vi "Check If Pixels Belong In Sector.vi"() -> (3 "FIFO Timeout?":bool)   [LabVIEW 2013]
uses:
  Single Sector Pixel Cluster.ctl
  Globals/Sector Parameter Global.vi
  Globals/Pixel Location Global.vi
  <vilib>/rvi/FIFO/Fifo_Resource/nirvififoEmulationReadFpgaImpl.vi
  <vilib>/rvi/DataTransferAndStorage/Container/Common/niFpgaContainerGetUniqueNameForEmu.vi
  <vilib>/rvi/FIFO/Fifo_Resource/nirvififoEmulationWriteFpgaImpl.vi
  <vilib>/rvi/DataTransferAndStorage/Container/XNode/niFpgaContainer.xnode
  <vilib>/rvi/FIFO/Fifo_Resource/nirvififoEmulationRead.vi
  <vilib>/rvi/FIFO/Fifo_Resource/nirvififoEmulationWrite.vi
panel:
  out "End of  Data?":bool
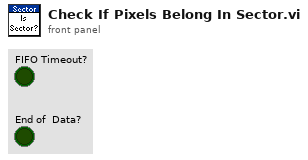
[diagram p1: front panel]
types:
  T1 = typedef "Single Sector Pixel Cluster.ctl" = cluster{"Sector #":u8, "Pixel Value":u8}
  T2 = typedef "Sector Parameter Cluster.ctl" = cluster{"Start Angle":fxp<+/-,17,2>, "End Angle":fxp<+/-,17,2>, "Inner Radius":u16, "Outter Radius":u16, "Hinge X":u16, "Hinge Y":u16, "NumWingSectors":u8}
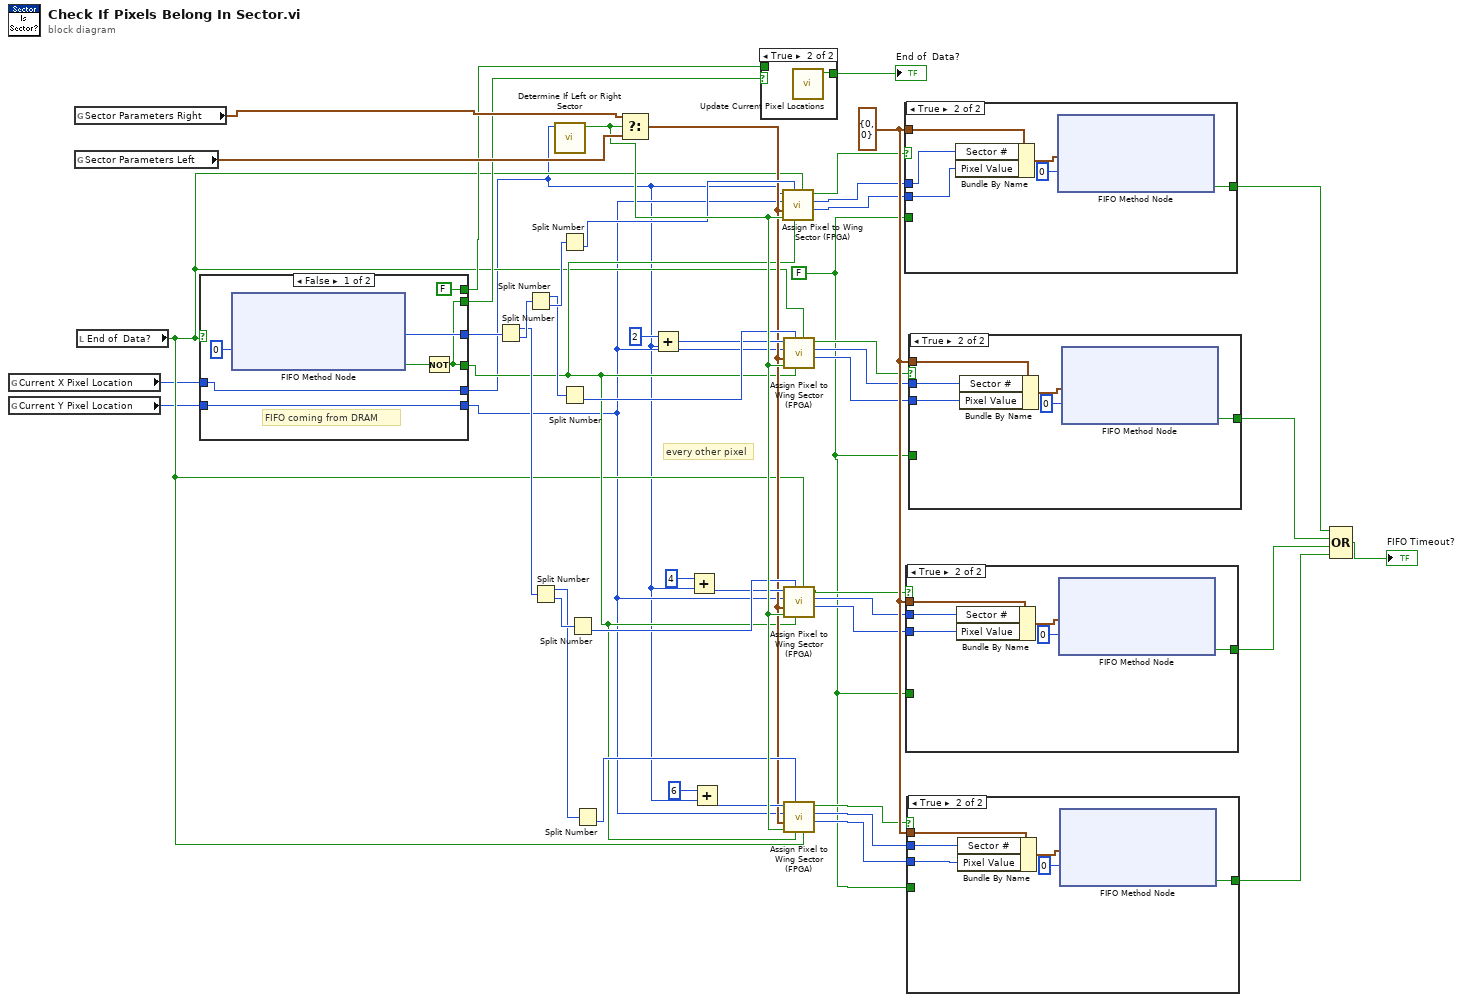
[diagram p0: block diagram]
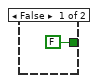
[diagram p3: hidden frame]
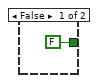
[diagram p4: hidden frame]
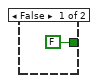
[diagram p5: hidden frame]
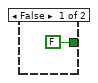
[diagram p6: hidden frame]
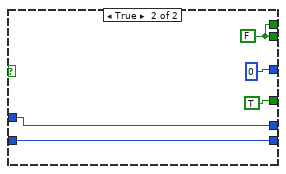
[diagram p7: hidden frame]
diagram:
  w27 = FALSE
  w40 = T1 {"Sector #"=0, "Pixel Value"=0} ("Single Sector Pixel")
  # "every other pixel"
  n1 = global read "Pixel Location Global.vi" "Current X Pixel Location"() -> (w1:u16)
  n2 = global read "Pixel Location Global.vi" "Current Y Pixel Location"() -> (w3:u16)
  n3 = global read "Sector Parameter Global.vi" "Sector Parameters Right"() -> (w47:T2)
  n4 = global read "Sector Parameter Global.vi" "Sector Parameters Left"() -> (w46:T2)
  n5 = local read "End of  Data?"() -> (w5:bool)
  n6 = case shown="False" w5 {
    tunnel: [w53 TRUE ("Timed Out?")] -> w8
    tunnel: [w55 u64 0 ("Element")] -> w45
    tunnel: [w53 w59] -> w7
    tunnel: [FALSE ("Timed Out?") w59] -> w6
    tunnel: [w51 w57] -> w4
    tunnel: w3 -> [w51 w57]
    tunnel: [w50 w58] -> w2
    tunnel: w1 -> [w50 w58]
    frame False {
      # "FIFO coming from DRAM"
      n7 = xnode ("FIFO Method Node")("Timeout"=0) -> ("Element"=w55:u64, "Timed Out?"=w54:bool)  [unwired: 1 in, 1 out]
      n8 = Not(x=w54) -> (.not. x?=w53:bool)
    }
    frame True {
      w59 = FALSE ("Timed Out?")
    }
  }
  n9 = Split Number(x=w45) -> (hi(x)=w25:u32, lo(x)=w26:u32)
  n10 = Split Number(x=w26) -> (hi(x)=w23:u16, lo(x)=w24:u16)
  n11 = Split Number(x=w25) -> (hi(x)=w21:u16, lo(x)=w22:u16)
  n12 = call "Determine If Left or Right Sector.vi"("X Pixel Location"=w2) -> ("Right Sector?"=w20:bool)  [unwired: 10 in]
  n13 = Split Number(x=w24) -> (lo(x)=w19:u8)  [unwired: 1 out]
  n14 = Split Number(x=w23) -> (lo(x)=w18:u8)  [unwired: 1 out]
  n15 = Split Number(x=w22) -> (lo(x)=w17:u8)  [unwired: 1 out]
  n16 = Split Number(x=w21) -> (lo(x)=w16:u8)  [unwired: 1 out]
  n17 = Select(t=w47, s=w20, f=w46) -> (s? t:f=w9:T2)
  n18 = Add(x=u16 2, y=w2) -> (x+y=w12:u16)
  n19 = Add(x=u16 4, y=w2) -> (x+y=w11:u16)
  n20 = Add(x=u16 6, y=w2) -> (x+y=w10:u16)
  n21 = case shown="True" w7 {
    tunnel: [w62 w63] -> w49
    tunnel: w6 -> [w62 _]
    frame False {
    }
    frame True {
      n22 = call "Update Current Pixel Locations.vi"() -> ("End of data?"=w63:bool)  [unwired: 11 in]
    }
  }
  "End of  Data?" <- w49
  n23 = call "Assign Pixel to Wing Sector (FPGA).vi"("End of Data?"=w5, "Valid Data?"=w8, "Pixel Intensity In"=w19, "Right Wing?"=w20, "Sector Parameters"=w9, "Pixel Y"=w4, "Pixel X"=w2) -> ("Pixel Intensity Out"=w37:u8, "sector #"=w38:u8, "output valid"=w39:bool)  [unwired: 2 out]
  n24 = call "Assign Pixel to Wing Sector (FPGA).vi"("End of Data?"=w5, "Valid Data?"=w8, "Pixel Intensity In"=w18, "Right Wing?"=w20, "Sector Parameters"=w9, "Pixel Y"=w4, "Pixel X"=w12) -> ("Pixel Intensity Out"=w34:u8, "sector #"=w35:u8, "output valid"=w36:bool)  [unwired: 2 out]
  n25 = call "Assign Pixel to Wing Sector (FPGA).vi"("End of Data?"=w5, "Valid Data?"=w8, "Pixel Intensity In"=w17, "Right Wing?"=w20, "Sector Parameters"=w9, "Pixel Y"=w4, "Pixel X"=w11) -> ("Pixel Intensity Out"=w31:u8, "sector #"=w32:u8, "output valid"=w33:bool)  [unwired: 2 out]
  n26 = call "Assign Pixel to Wing Sector (FPGA).vi"("End of Data?"=w5, "Valid Data?"=w8, "Pixel Intensity In"=w16, "Right Wing?"=w20, "Sector Parameters"=w9, "Pixel Y"=w4, "Pixel X"=w10) -> ("Pixel Intensity Out"=w28:u8, "sector #"=w29:u8, "output valid"=w30:bool)  [unwired: 2 out]
  n27 = case shown="True" w39 {
    tunnel: w40 -> [_ w65]
    tunnel: [FALSE ("Timed Out?") w68] -> w44
    tunnel: w38 -> [_ w66]
    tunnel: w37 -> [_ w67]
    tunnel: w27 -> [_ _]
    frame False {
    }
    frame True {
      n28 = Bundle By Name(cluster=w65, "Sector #"=w66, "Pixel Value"=w67) -> (w69:T1)
      n29 = xnode ("FIFO Method Node")("Element"=w69, "Timeout"=0) -> ("Timed Out?"=w68:bool)  [unwired: 1 in, 1 out]
    }
  }
  n30 = case shown="True" w33 {
    tunnel: w40 -> [_ w77]
    tunnel: [FALSE ("Timed Out?") w74] -> w42
    tunnel: w32 -> [_ w72]
    tunnel: w31 -> [_ w73]
    tunnel: w27 -> [_ _]
    frame False {
    }
    frame True {
      n31 = Bundle By Name(cluster=w77, "Sector #"=w72, "Pixel Value"=w73) -> (w75:T1)
      n32 = xnode ("FIFO Method Node")("Element"=w75, "Timeout"=0) -> ("Timed Out?"=w74:bool)  [unwired: 1 in, 1 out]
    }
  }
  n33 = case shown="True" w30 {
    tunnel: w40 -> [_ w84]
    tunnel: [FALSE ("Timed Out?") w81] -> w41
    tunnel: w29 -> [_ w79]
    tunnel: w28 -> [_ w80]
    tunnel: w27 -> [_ _]
    frame False {
    }
    frame True {
      n34 = Bundle By Name(cluster=w84, "Sector #"=w79, "Pixel Value"=w80) -> (w82:T1)
      n35 = xnode ("FIFO Method Node")("Element"=w82, "Timeout"=0) -> ("Timed Out?"=w81:bool)  [unwired: 1 in, 1 out]
    }
  }
  n36 = case shown="True" w36 {
    tunnel: w40 -> [_ w91]
    tunnel: [FALSE ("Timed Out?") w88] -> w43
    tunnel: w35 -> [_ w86]
    tunnel: w34 -> [_ w87]
    tunnel: w27 -> [_ _]
    frame False {
    }
    frame True {
      n37 = Bundle By Name(cluster=w91, "Sector #"=w86, "Pixel Value"=w87) -> (w89:T1)
      n38 = xnode ("FIFO Method Node")("Element"=w89, "Timeout"=0) -> ("Timed Out?"=w88:bool)  [unwired: 1 in, 1 out]
    }
  }
  n39 = Compound Arithmetic op=OR(w44, w43, w42, w41) -> (→"FIFO Timeout?":bool)
